vi "SetHome.vi"(2 "error in (no error)":errorcluster, 3 "StepperController in":refnum<class "StepperController.lvclass">) -> (0 "error out":errorcluster, 1 "StepperController out":refnum<class "StepperController.lvclass">)   [LabVIEW 2013, in "StepperController.lvclass"]
uses:
  StepperController.lvclass
  StepperController.lvclass/StepperController.ctl
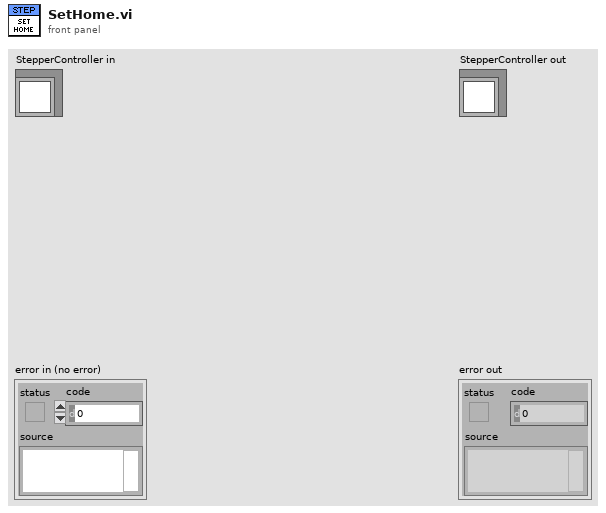
[diagram p1: front panel]
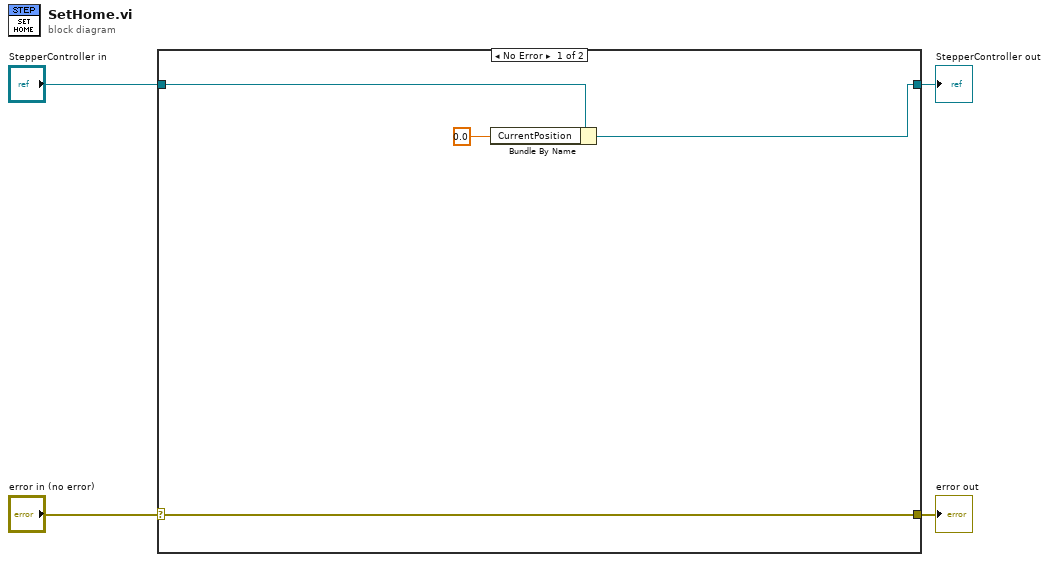
[diagram p0: block diagram]
diagram:
  n1 = case shown="No Error" "error in (no error)" {
    selector: "error in (no error)" -> [w8 w9]
    tunnel: [w8 w9] -> w3
    tunnel: [w6 w10] -> w1
    tunnel: "StepperController in" -> [w7 w10]
    frame No Error {
      n2 = Bundle By Name(cluster=w7, "CurrentPosition"=0.0) -> (w6:refnum<class "StepperController.lvclass">)
    }
    frame Error {
    }
  }
  "error out" <- w3
  "StepperController out" <- w1
